vi "PCA Read.vi"(8 "error in (no error)":errorcluster, 10 "File Path":path, 11 "PCA in":refnum<class "PCA.lvclass">) -> (0 "error out":errorcluster, 3 "PCA out":refnum<class "PCA.lvclass">)   [LabVIEW 2020, in "OpenLvVision_OpenCv.lvlib" / "PCA.lvclass"]
doc: "Loads eigenvalues eigenvectors and mean from specified FileNode"
uses:
  PCA.lvclass
  C:/Users/lukas/Downloads/OpenLvVision_OpenCv/SourceCode/LabView/OpenLvVision_OpenCv/_LvHelpers/EdvrObject/EdvrObject.lvclass
  _LvHelpers/EdvrObject/EdvrObject.lvclass/EdvrObject.ctl
  _LvHelpers/EdvrObject/EdvrObject.lvclass
  Dlls/OlvOpenCvWrapper.dll
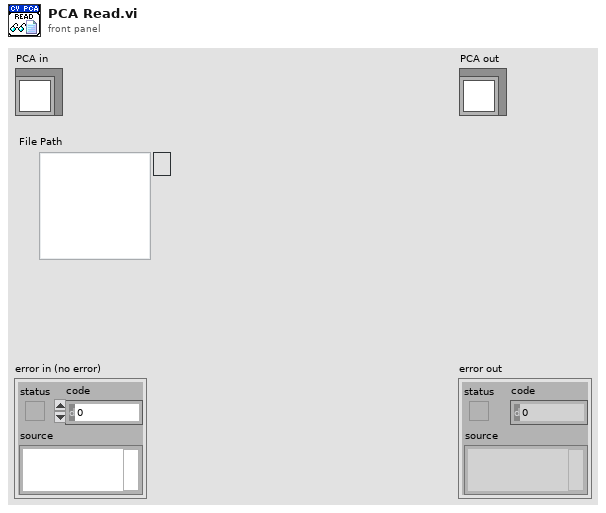
[diagram p1: front panel]
types:
  T1 = typedef "OpenLvVision_OpenCv.lvlib/EdvrObject.lvclass/Edvr.ctl" = refnum<data-value>
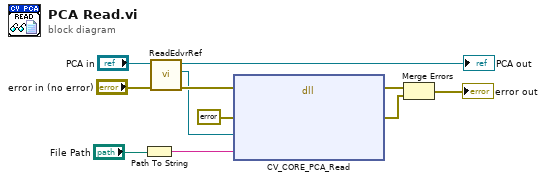
[diagram p0: block diagram]
diagram:
  n1 = Path To String(path="File Path") -> (string=w1:string)
  n2 = call "ReadEdvrRef.vi"("error in (no error)"="error in (no error)", "EdvrObject in"="PCA in") -> ("error out"=w11:errorcluster, "Edvr"=w10:T1, "EdvrObject out"=→"PCA out":refnum<class "PCA.lvclass">)  [unwired: 7 in]
  n3 = dll-call lib="C:/Users/lukas/Downloads/OpenLvVision_OpenCv/SourceCode/LabView/OpenLvVision_OpenCv/Dlls/OlvOpenCvWrapper.dll" fn="CV_CORE_PCA_Read"(error in=w11, "Error"=errorcluster {"status"=FALSE, "code"=0, "source"=""}, "edvrRef"=w10, "filePath"=w1) -> (error out=w8:errorcluster, "Error"=w7:errorcluster)  [unwired: 5 in, 1 out]
  n4 = Merge Errors(w8, w7) -> (→"error out":errorcluster)
